vi "gm_measuringmode.vi"(9 "rt_vars in":T2, 10 "Output - Cluster gas in":T1 {"GM TS-2[°C]" format="%.2g"; "GM TS-1 [°C]" format="%.2g"; "GM DS-1 [bar]" format="%.4g"; "GM DS-2 [bar]" format="%.4g"; "GA1 h2 [%]" format="%.2g"; "GA1 co2 [%]" format="%.2g"; "GA1 ch4 [%]" format="%.2g"}, 11 "Input - Cluster gas in":T3) -> (1 "rt_vars out":T2, 2 "Output - Cluster gas out":T1 {"GM TS-2[°C]" format="%.2g"; "GM TS-1 [°C]" format="%.2g"; "GM DS-1 [bar]" format="%.4g"; "GM DS-2 [bar]" format="%.4g"; "GA1 h2 [%]" format="%.2g"; "GA1 co2 [%]" format="%.2g"; "GA1 ch4 [%]" format="%.2g"}, 3 "Input - Cluster gas out":T3)   [LabVIEW 2011]
uses:
  Input - Cluster gas.ctl
  Output - Cluster gas.ctl
panel:
  # "converted bool array!"
  # "mode :\n0: nothing\n1: quality\n2: quantity\n3: quality and quantity"
  # "converted bool array!"
  # "mode :\n0: nothing\n1: quality\n2: quantity\n3: quality and quantity"
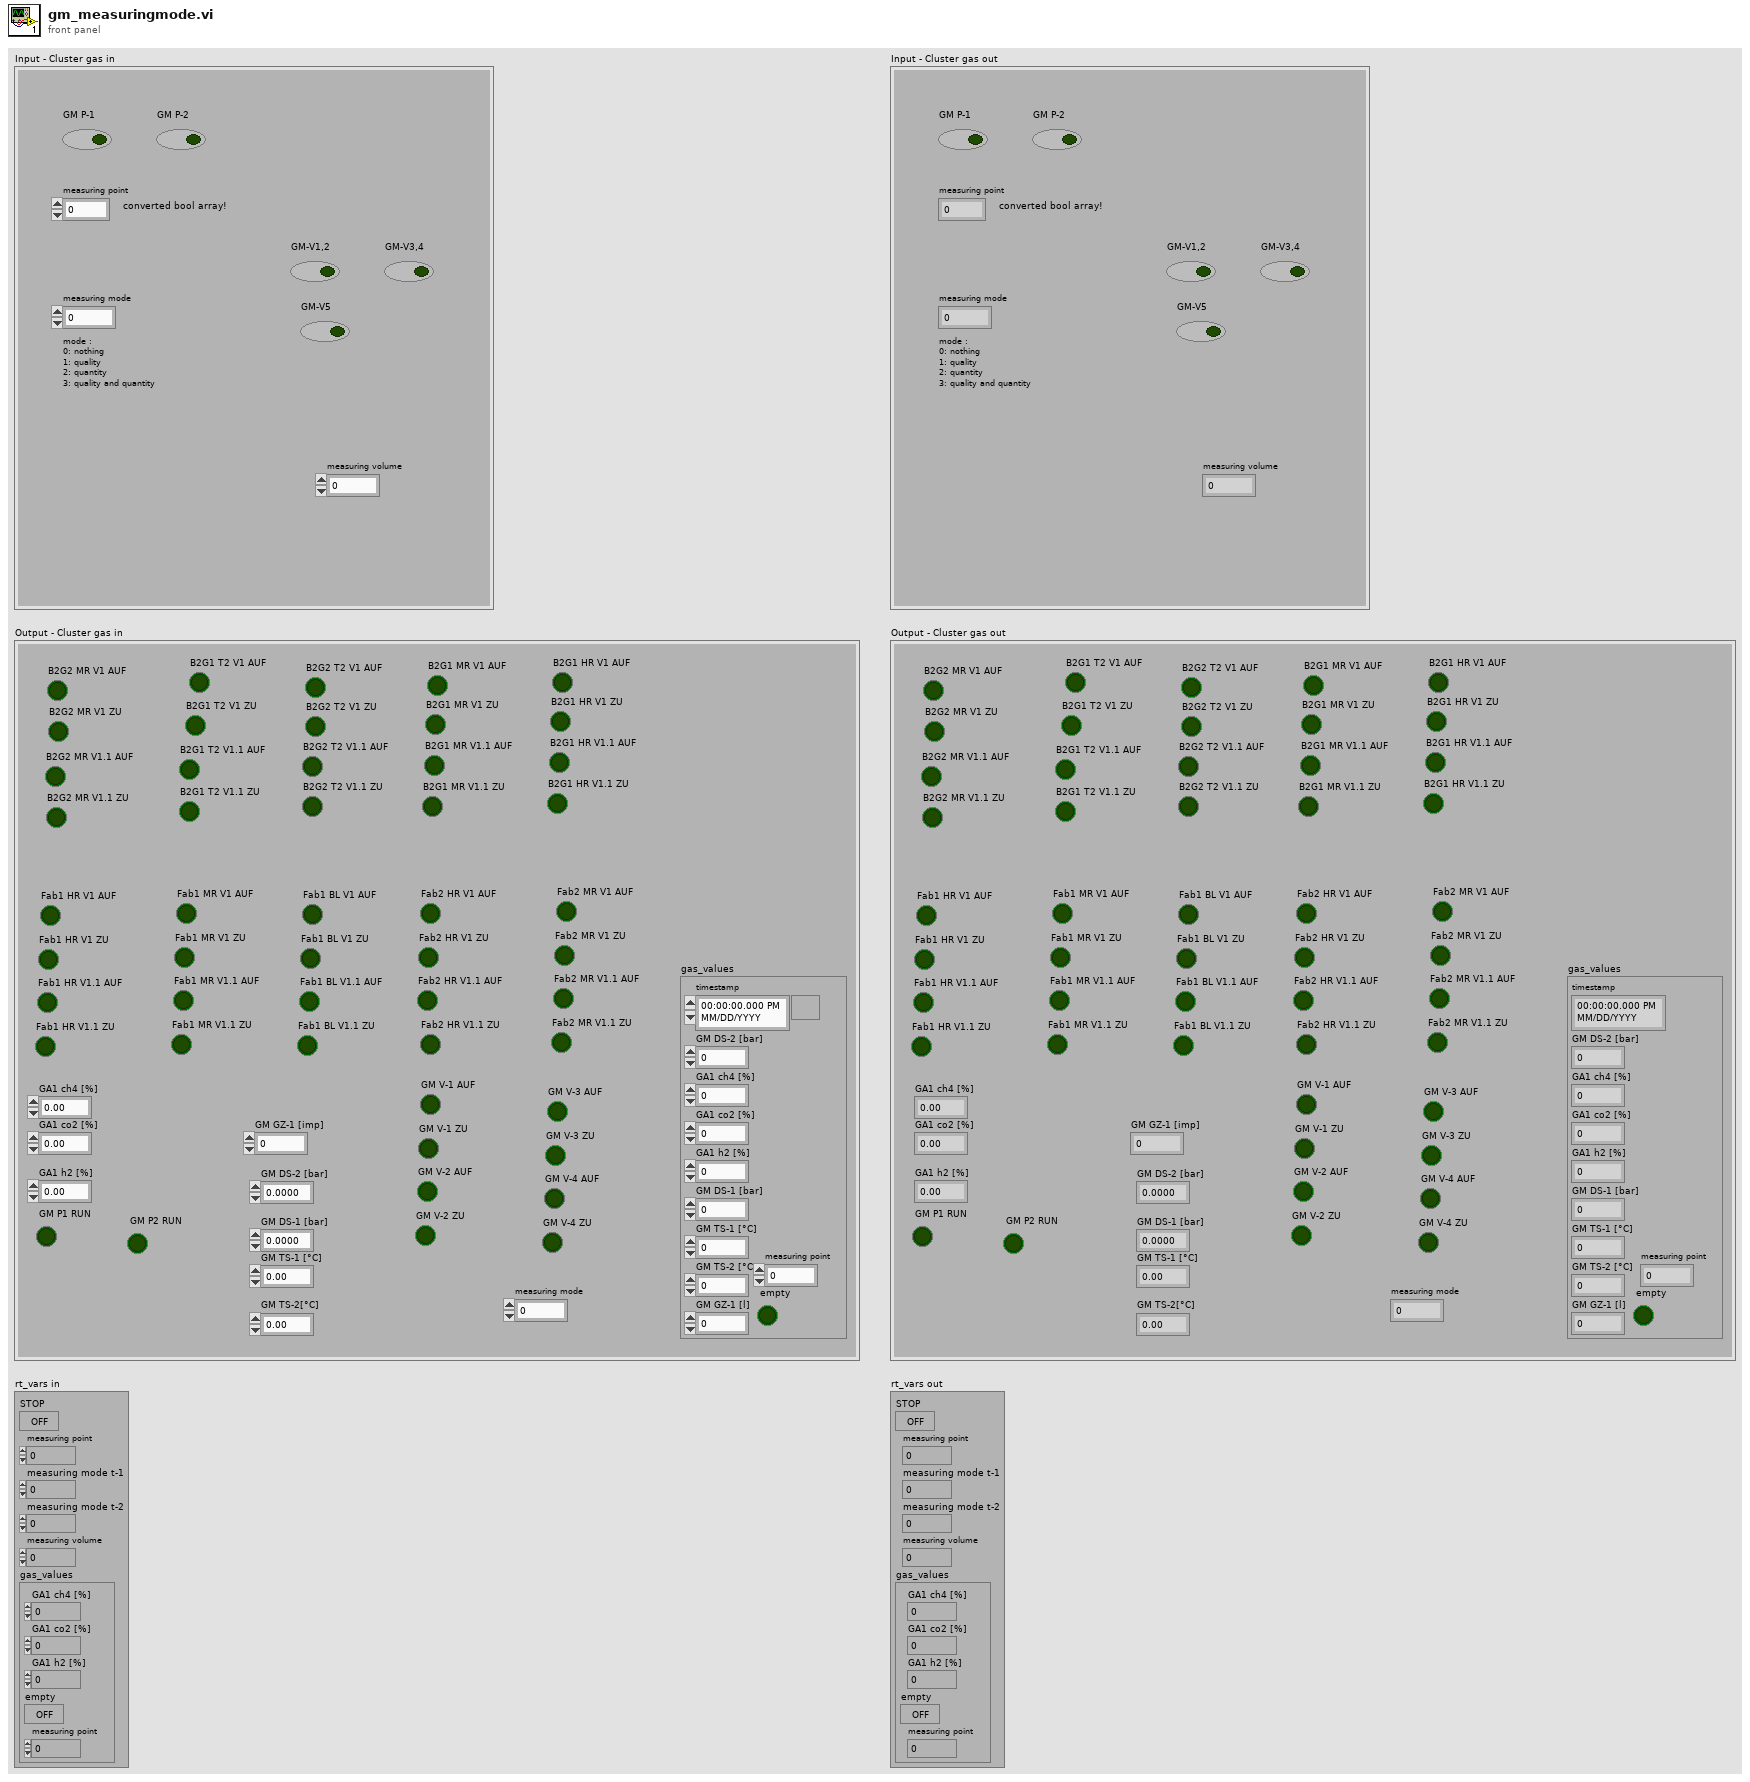
[diagram p1: front panel]
types:
  T1 = typedef "Output - Cluster gas.ctl" = cluster{"B2G2 MR V1.1 AUF":bool, "B2G2 MR V1.1 ZU":bool, "B2G2 MR V1 AUF":bool, "B2G2 MR V1 ZU":bool, "B2G1 T2 V1 AUF":bool, "B2G1 T2 V1 ZU":bool, "B2G1 T2 V1.1 AUF":bool, "B2G1 T2 V1.1 ZU":bool, "B2G2 T2 V1 AUF":bool, "B2G2 T2 V1 ZU":bool, "B2G2 T2 V1.1 ZU":bool, "B2G2 T2 V1.1 AUF":bool, "B2G1 MR V1 AUF":bool, "B2G1 MR V1 ZU":bool, "B2G1 MR V1.1 AUF":bool, "B2G1 MR V1.1 ZU":bool, "B2G1 HR V1 AUF":bool, "B2G1 HR V1 ZU":bool, "B2G1 HR V1.1 AUF":bool, "B2G1 HR V1.1 ZU":bool, "Fab1 HR V1 AUF":bool, "Fab1 HR V1 ZU":bool, "Fab1 HR V1.1 AUF":bool, "Fab1 HR V1.1 ZU":bool, "Fab1 MR V1 AUF":bool, "Fab1 MR V1 ZU":bool, "Fab1 MR V1.1 AUF":bool, "Fab1 MR V1.1 ZU":bool, "Fab1 BL V1 AUF":bool, "Fab1 BL V1 ZU":bool, "Fab1 BL V1.1 AUF":bool, "Fab1 BL V1.1 ZU":bool, "Fab2 HR V1 AUF":bool, "Fab2 HR V1 ZU":bool, "Fab2 HR V1.1 AUF":bool, "Fab2 HR V1.1 ZU":bool, "Fab2 MR V1 AUF":bool, "Fab2 MR V1 ZU":bool, "Fab2 MR V1.1 AUF":bool, "Fab2 MR V1.1 ZU":bool, "GA1 ch4 [%]":dbl, "GA1 co2 [%]":dbl, "GA1 h2 [%]":dbl, "GM P1 RUN":bool, "GM V-1 AUF":bool, "GM V-1 ZU":bool, "GM V-2 AUF":bool, "GM V-2 ZU":bool, "GM V-3 AUF":bool, "GM V-3 ZU":bool, "GM V-4 AUF":bool, "GM V-4 ZU":bool, "GM P2 RUN":bool, "GM GZ-1 [imp]":u32, "GM DS-2 [bar]":dbl, "GM DS-1 [bar]":dbl, "GM TS-1 [°C]":dbl, "GM TS-2[°C]":dbl, "gas_values":cluster{"timestamp":timestamp, "GM DS-2 [bar]":dbl, "GA1 ch4 [%]":dbl, "GA1 co2 [%]":dbl, "GA1 h2 [%]":dbl, "GM DS-1 [bar]":dbl, "GM TS-1 [°C]":dbl, "GM TS-2 [°C]":dbl, "GM GZ-1 [l]":dbl, "empty":bool, "measuring point":u8}, "measuring mode":u8}
  T2 = cluster{"STOP":bool, "measuring point":u32, "measuring mode t-1":u8, "measuring mode t-2":u8, "measuring volume":u32, "gas_values":cluster{"GA1 ch4 [%]":dbl, "GA1 co2 [%]":dbl, "GA1 h2 [%]":dbl, "empty":bool, "measuring point":u8}}
  T3 = typedef "Input - Cluster gas.ctl" = cluster{"GM P-1":bool, "GM P-2":bool, "measuring point":u32, "measuring mode":u8, "GM-V1,2":bool, "GM-V3,4":bool, "GM-V5":bool, "measuring volume":u32}
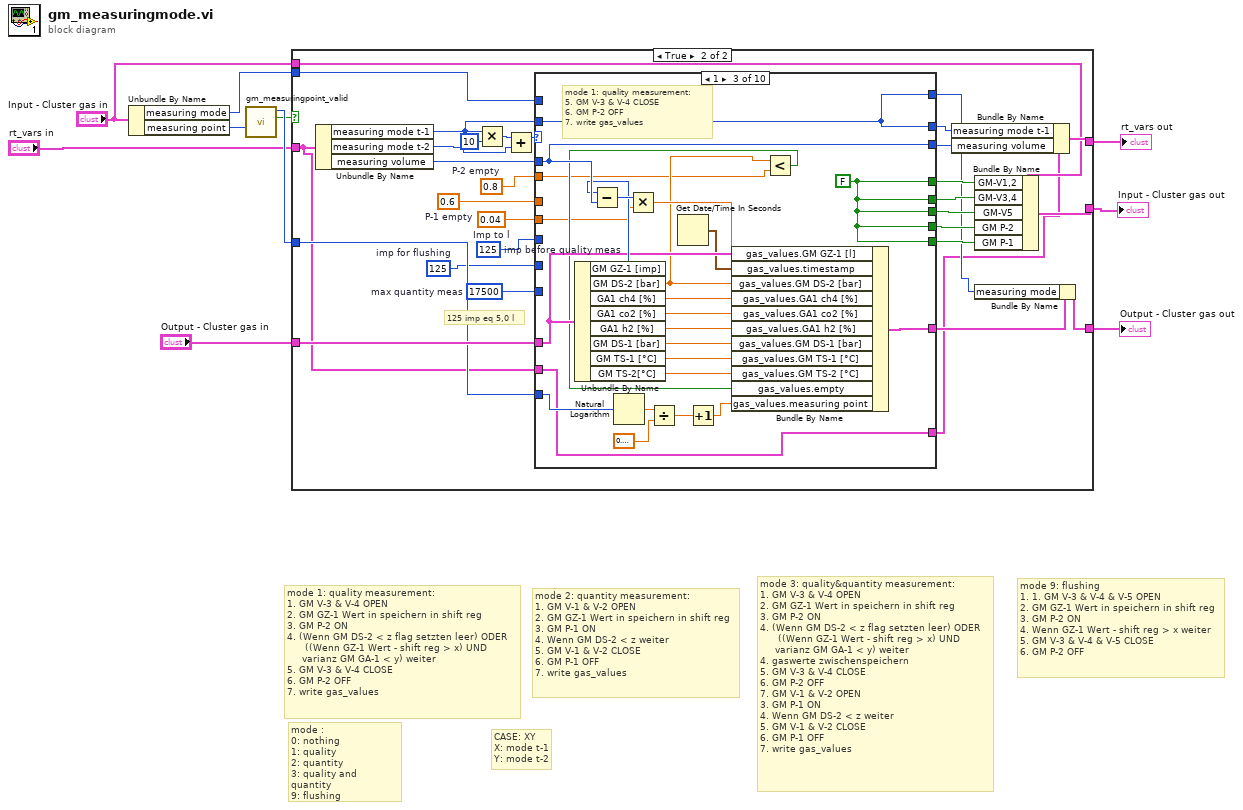
[diagram p0: block diagram]
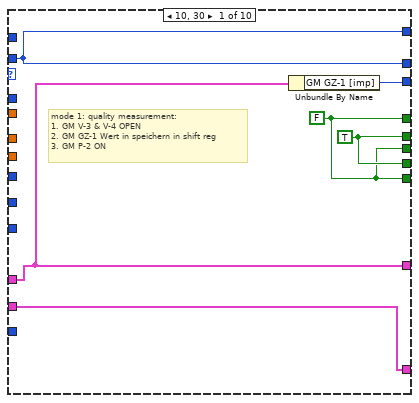
[diagram p3: hidden frame]
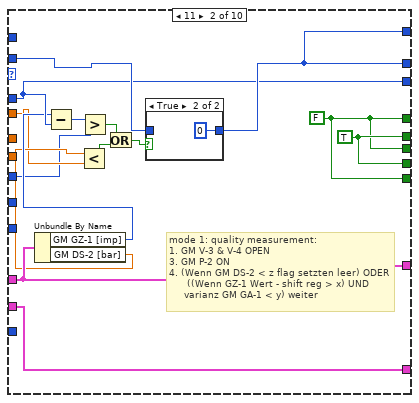
[diagram p4: hidden frame]
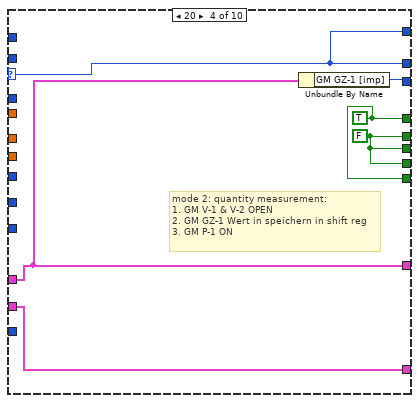
[diagram p6: hidden frame]
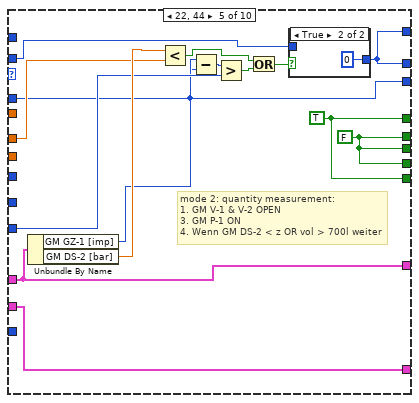
[diagram p7: hidden frame]
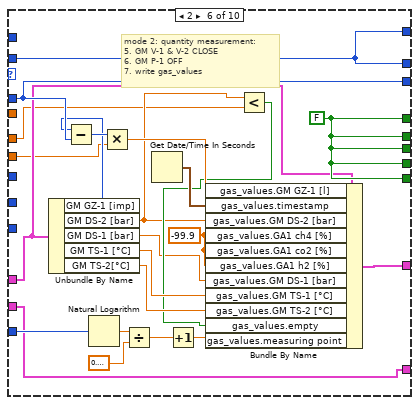
[diagram p9: hidden frame]
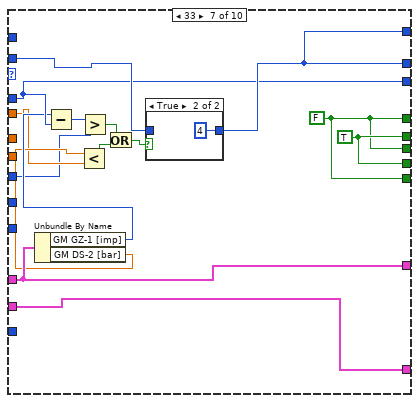
[diagram p10: hidden frame]
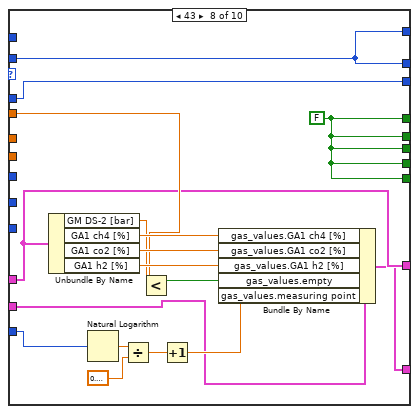
[diagram p12: hidden frame]
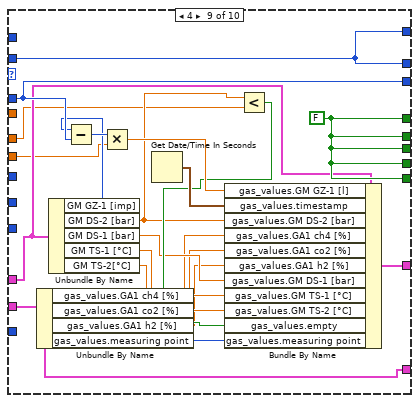
[diagram p13: hidden frame]
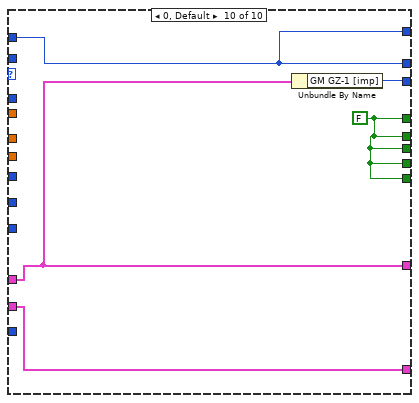
[diagram p14: hidden frame]
diagram:
  # "mode :\n0: nothing\n1: quality\n2: quantity\n3: quality and quantity\n9: flushing"
  # "mode 9: flushing\n1. 1. GM V-3 & V-4 & V-5 OPEN\n2. GM GZ-1 Wert in speichern in shift reg\n3. GM P-2 ON\n4. Wenn GZ-1 Wert - shift reg > x weiter \n5. GM V-3 & V-4 & V-5 CLOSE\n6. GM P-2 OFF"
  # "CASE: XY\nX: mode t-1\nY: mode t-2"
  # "mode 3: quality&quantity measurement:\n1. GM V-3 & V-4 OPEN\n2. GM GZ-1 Wert in speichern in shift reg\n3. GM P-2 ON\n4. (Wenn GM DS-2 < z flag setzten leer) ODER\n      ((Wenn GZ-1 Wert - shift reg > x) UND\n     varianz GM GA-1 < y) weiter\n4. gaswerte zwischenspeichern\n5. GM V-3 & V-4 CLOSE\n6. GM P-2 OFF\n7. GM V-1 & V-2 OPEN\n3. GM P-1 ON\n4. Wenn GM DS-2 < z weiter\n5. GM V-1 & V-2 CLOSE\n6. GM P-1 OFF\n7. write gas_values"
  # "mode 2: quantity measurement:\n1. GM V-1 & V-2 OPEN\n2. GM GZ-1 Wert in speichern in shift reg\n3. GM P-1 ON\n4. Wenn GM DS-2 < z weiter\n5. GM V-1 & V-2 CLOSE\n6. GM P-1 OFF\n7. write gas_values"
  # "mode 1: quality measurement:\n1. GM V-3 & V-4 OPEN\n2. GM GZ-1 Wert in speichern in shift reg\n3. GM P-2 ON\n4. (Wenn GM DS-2 < z flag setzten leer) ODER\n      ((Wenn GZ-1 Wert - shift reg > x) UND\n     varianz GM GA-1 < y) weiter\n5. GM V-3 & V-4 CLOSE\n6. GM P-2 OFF\n7. write gas_values"
  n1 = Unbundle By Name("Input - Cluster gas in") -> ("measuring mode"=w3:u8, "measuring point"=w2:u32)
  n2 = call "gm_measuringpoint_valid.vi"("measuring point in"=w2) -> ("Boolean"=w1:bool, "measuring point out"=w10:u32)  [unwired: 9 in]
  n3 = case shown="True" w1 {
    tunnel: w3 -> [_ w43]
    tunnel: "Output - Cluster gas in" -> [w13 w39]
    tunnel: [w13 w24] -> w5
    tunnel: "rt_vars in" -> [w12 w16]
    tunnel: [w12 w35] -> w7
    tunnel: "Input - Cluster gas in" -> [w11 w27]
    tunnel: [w11 w26] -> w9
    tunnel: w10 -> [_ w22]
    frame False {
    }
    frame True {
      w14 = u32 125  # imp for flushing
      w17 = u32 17500  # max quantity meas
      w18 = u32 125  # imp before quality meas
      w19 = 0.6  # P-1 empty
      w20 = 0.8  # P-2 empty
      w21 = 0.04  # Imp to l
      # "125 imp eq 5,0 l"
      n4 = Unbundle By Name(w16) -> ("measuring mode t-1"=w38:u8, "measuring mode t-2"=w37:u8, "measuring volume"=w36:u32)
      n5 = Multiply(x=w38, y=u8 10) -> (x*y=w42:u8)
      n6 = Add(x=w42, y=w37) -> (x+y=w41:u8)
      n7 = case shown="1" w41 {
        selector: w41 -> [_ _ _ w97 _ _ _ _ _ _]
        tunnel: w43 -> [_ _ _ _ _ _ _ _ _ w197]
        tunnel: [w48 w61 w90 w97 w110 w136 w149 w170 w191 w197] -> w34
        tunnel: [w44 w63 w91 w96 w112 w137 w151 w171 w192 w196] -> w32
        tunnel: [w49 w64 w91 w95 w107 w137 w152 w171 w192 w196] -> w31
        tunnel: [w44 w63 w91 w95 w107 w137 w151 w171 w192 w196] -> w30
        tunnel: [w48 w61 w90 w97 w110 w136 w149 w170 w191 w197] -> w23
        tunnel: [w46 w60 w89 w93 w100 w135 w148 w169 w190 w194] -> w33
        tunnel: [w49 w64 w91 w95 w107 w137 w152 w171 w192 w196] -> w29
        tunnel: [w44 w63 w91 w96 w112 w137 w151 w171 w192 w196] -> w28
        tunnel: w36 -> [_ w60 w89 _ w100 w135 w148 w169 w190 _]
        tunnel: w38 -> [w48 w62 w90 _ w111 w136 w150 w170 w191 _]
        tunnel: w39 -> [w47 w55 w85 w94 w109 w131 w143 w157 w186 w195]
        tunnel: [w47 w55 w86 w94 w109 w132 w143 w157 w187 w195] -> w25
        tunnel: w22 -> [_ _ w74 _ _ w120 _ w162 _ _]
        tunnel: w21 -> [_ _ w69 _ _ w116 _ _ w177 _]
        tunnel: w20 -> [_ w52 w68 _ _ _ w140 w158 _ _]
        tunnel: w19 -> [_ _ _ _ w106 w117 _ _ w178 _]
        tunnel: w18 -> [_ w51 _ _ _ _ w139 _ _ _]
        tunnel: w17 -> [_ _ _ _ w102 _ _ _ _ _]
        tunnel: w16 -> [w45 w50 w67 w92 w98 w115 w138 w156 w176 w193]
        tunnel: [w45 w50 w67 w92 w98 w115 w138 w155 w176 w193] -> w15
        tunnel: w14 -> [_ _ _ _ _ _ _ _ _ _]
        frame 10, 30 {
          w44 = FALSE ("GM-V3,4")
          w49 = TRUE ("GM-V3,4")
          # "mode 1: quality measurement:\n1. GM V-3 & V-4 OPEN\n2. GM GZ-1 Wert in speichern in shift reg\n3. GM P-2 ON"
          n8 = Unbundle By Name(w47) -> ("GM GZ-1 [imp]"=w46:u32)
        }
        frame 11 {
          w63 = FALSE ("GM-V3,4")
          w64 = TRUE ("GM-V3,4")
          # "mode 1: quality measurement:\n1. GM V-3 & V-4 OPEN\n3. GM P-2 ON\n4. (Wenn GM DS-2 < z flag setzten leer) ODER\n      ((Wenn GZ-1 Wert - shift reg > x) UND\n     varianz GM GA-1 < y) weiter"
          n9 = Unbundle By Name(w55) -> ("GM GZ-1 [imp]"=w54:u32, "GM DS-2 [bar]"=w53:dbl)
          n10 = Subtract(x=w54, y=w60) -> (x-y=w59:u32)
          n11 = Less?(x=w53, y=w52) -> (x < y?=w56:bool)
          n12 = Greater?(x=w59, y=w51) -> (0:w57:bool)
          n13 = Or(x=w57, y=w56) -> (x .or. y?=w58:bool)
          n14 = case shown="True" w58 {
            tunnel: w62 -> [w65 _]
            tunnel: [w65 u8 0 ("measuring mode t-1")] -> w61
            frame False {
            }
            frame True {
            }
          }
        }
        frame 1 {
          w91 = FALSE ("GM-V3,4")
          # "mode 1: quality measurement:\n5. GM V-3 & V-4 CLOSE\n6. GM P-2 OFF\n7. write gas_values"
          n15 = Unbundle By Name(w85) -> ("GM GZ-1 [imp]"=w87:u32, "GM DS-2 [bar]"=w71:dbl, "GA1 ch4 [%]"=w82:dbl, "GA1 co2 [%]"=w81:dbl, "GA1 h2 [%]"=w80:dbl, "GM DS-1 [bar]"=w70:dbl, "GM TS-1 [°C]"=w79:dbl, "GM TS-2[°C]"=w78:dbl)
          n16 = Subtract(x=w87, y=w89) -> (x-y=w88:u32)
          n17 = Natural Logarithm(1:w74) -> (0:w76:dbl)
          n18 = Multiply(x=w88, y=w69) -> (x*y=w83:dbl)
          n19 = Divide(x=w76, y=0.6931471805599453) -> (x/y=w73:dbl)
          n20 = Get Date/Time In Seconds ("timestamp")() -> (seconds since 1Jan1904=w84:timestamp)
          n21 = Increment(x=w73) -> (x+1=w72:dbl)
          n22 = Less?(x=w71, y=w68) -> (x < y?=w77:bool)
          n23 = Bundle By Name(cluster=w85, "gas_values.GM GZ-1 [l]"=w83, "gas_values.timestamp"=w84, "gas_values.GM DS-2 [bar]"=w71, "gas_values.GA1 ch4 [%]"=w82, "gas_values.GA1 co2 [%]"=w81, "gas_values.GA1 h2 [%]"=w80, "gas_values.GM DS-1 [bar]"=w70, "gas_values.GM TS-1 [°C]"=w79, "gas_values.GM TS-2 [°C]"=w78, "gas_values.empty"=w77, "gas_values.measuring point"=w72) -> (w86:T1)
        }
        frame 20 {
          w95 = FALSE ("GM-V3,4")
          w96 = TRUE ("GM-V3,4")
          # "mode 2: quantity measurement:\n1. GM V-1 & V-2 OPEN\n2. GM GZ-1 Wert in speichern in shift reg\n3. GM P-1 ON"
          n24 = Unbundle By Name(w94) -> ("GM GZ-1 [imp]"=w93:u32)
        }
        frame 22, 44 {
          w112 = TRUE ("GM-V3,4")
          w107 = FALSE ("GM-V3,4")
          # "mode 2: quantity measurement:\n1. GM V-1 & V-2 OPEN\n3. GM P-1 ON\n4. Wenn GM DS-2 < z OR vol > 700l weiter"
          n25 = Unbundle By Name(w109) -> ("GM GZ-1 [imp]"=w101:u32, "GM DS-2 [bar]"=w108:dbl)
          n26 = Less?(x=w108, y=w106) -> (x < y?=w105:bool)
          n27 = Subtract(x=w101, y=w100) -> (x-y=w103:u32)
          n28 = Greater?(x=w103, y=w102) -> (0:w99:bool)
          n29 = Or(x=w105, y=w99) -> (x .or. y?=w104:bool)
          n30 = case shown="True" w104 {
            tunnel: w111 -> [w113 _]
            tunnel: [w113 u8 0 ("measuring mode t-1")] -> w110
            frame False {
            }
            frame True {
            }
          }
        }
        frame 2 {
          w125 = -99.9 ("gas_values.GA1 ch4 [%]")
          w137 = FALSE ("GM-V3,4")
          # "mode 2: quantity measurement:\n5. GM V-1 & V-2 CLOSE\n6. GM P-1 OFF\n7. write gas_values"
          n31 = Unbundle By Name(w131) -> ("GM GZ-1 [imp]"=w133:u32, "GM DS-2 [bar]"=w119:dbl, "GM DS-1 [bar]"=w118:dbl, "GM TS-1 [°C]"=w128:dbl, "GM TS-2[°C]"=w127:dbl)
          n32 = Subtract(x=w133, y=w135) -> (x-y=w134:u32)
          n33 = Natural Logarithm(1:w120) -> (0:w124:dbl)
          n34 = Multiply(x=w134, y=w116) -> (x*y=w129:dbl)
          n35 = Divide(x=w124, y=0.6931471805599453) -> (x/y=w122:dbl)
          n36 = Get Date/Time In Seconds ("timestamp")() -> (seconds since 1Jan1904=w130:timestamp)
          n37 = Increment(x=w122) -> (x+1=w121:dbl)
          n38 = Less?(x=w119, y=w117) -> (x < y?=w126:bool)
          n39 = Bundle By Name(cluster=w131, "gas_values.GM GZ-1 [l]"=w129, "gas_values.timestamp"=w130, "gas_values.GM DS-2 [bar]"=w119, "gas_values.GA1 ch4 [%]"=w125, "gas_values.GA1 co2 [%]"=w125, "gas_values.GA1 h2 [%]"=w125, "gas_values.GM DS-1 [bar]"=w118, "gas_values.GM TS-1 [°C]"=w128, "gas_values.GM TS-2 [°C]"=w127, "gas_values.empty"=w126, "gas_values.measuring point"=w121) -> (w132:T1)
        }
        frame 33 {
          w151 = FALSE ("GM-V3,4")
          w152 = TRUE ("GM-V3,4")
          n40 = Unbundle By Name(w143) -> ("GM GZ-1 [imp]"=w142:u32, "GM DS-2 [bar]"=w141:dbl)
          n41 = Subtract(x=w142, y=w148) -> (x-y=w147:u32)
          n42 = Less?(x=w141, y=w140) -> (x < y?=w144:bool)
          n43 = Greater?(x=w147, y=w139) -> (0:w145:bool)
          n44 = Or(x=w145, y=w144) -> (x .or. y?=w146:bool)
          n45 = case shown="True" w146 {
            tunnel: w150 -> [w153 _]
            tunnel: [w153 u8 4 ("measuring mode t-1")] -> w149
            frame False {
            }
            frame True {
            }
          }
        }
        frame 43 {
          w171 = FALSE ("GM-V3,4")
          n46 = Unbundle By Name(w157) -> ("GM DS-2 [bar]"=w159:dbl, "GA1 ch4 [%]"=w168:dbl, "GA1 co2 [%]"=w167:dbl, "GA1 h2 [%]"=w166:dbl)
          n47 = Natural Logarithm(1:w162) -> (0:w164:dbl)
          n48 = Divide(x=w164, y=0.6931471805599453) -> (x/y=w161:dbl)
          n49 = Less?(x=w159, y=w158) -> (x < y?=w165:bool)
          n50 = Increment(x=w161) -> (x+1=w160:dbl)
          n51 = Bundle By Name(cluster=w156, "gas_values.GA1 ch4 [%]"=w168, "gas_values.GA1 co2 [%]"=w167, "gas_values.GA1 h2 [%]"=w166, "gas_values.empty"=w165, "gas_values.measuring point"=w160) -> (w155:T2)
        }
        frame 4 {
          w192 = FALSE ("GM-V3,4")
          n52 = Unbundle By Name(w176) -> ("gas_values.GA1 ch4 [%]"=w174:dbl, "gas_values.GA1 co2 [%]"=w173:dbl, "gas_values.GA1 h2 [%]"=w172:dbl, "gas_values.measuring point"=w175:u8)
          n53 = Unbundle By Name(w186) -> ("GM GZ-1 [imp]"=w188:u32, "GM DS-2 [bar]"=w180:dbl, "GM DS-1 [bar]"=w179:dbl, "GM TS-1 [°C]"=w183:dbl, "GM TS-2[°C]"=w182:dbl)
          n54 = Subtract(x=w188, y=w190) -> (x-y=w189:u32)
          n55 = Multiply(x=w189, y=w177) -> (x*y=w184:dbl)
          n56 = Get Date/Time In Seconds ("timestamp")() -> (seconds since 1Jan1904=w185:timestamp)
          n57 = Less?(x=w180, y=w178) -> (x < y?=w181:bool)
          n58 = Bundle By Name(cluster=w186, "gas_values.GM GZ-1 [l]"=w184, "gas_values.timestamp"=w185, "gas_values.GM DS-2 [bar]"=w180, "gas_values.GA1 ch4 [%]"=w174, "gas_values.GA1 co2 [%]"=w173, "gas_values.GA1 h2 [%]"=w172, "gas_values.GM DS-1 [bar]"=w179, "gas_values.GM TS-1 [°C]"=w183, "gas_values.GM TS-2 [°C]"=w182, "gas_values.empty"=w181, "gas_values.measuring point"=w175) -> (w187:T1)
        }
        frame 0, Default {
          w196 = FALSE ("GM-V3,4")
          n59 = Unbundle By Name(w195) -> ("GM GZ-1 [imp]"=w194:u32)
        }
      }
      n60 = Bundle By Name(cluster=w15, "measuring mode t-1"=w34, "measuring volume"=w33) -> (w35:T2)
      n61 = Bundle By Name(cluster=w27, "GM-V1,2"=w32, "GM-V3,4"=w31, "GM-V5"=w30, "GM P-2"=w29, "GM P-1"=w28) -> (w26:T3)
      n62 = Bundle By Name(cluster=w25, "measuring mode"=w23) -> (w24:T1)
    }
  }
  "Input - Cluster gas out" <- w9
  "rt_vars out" <- w7
  "Output - Cluster gas out" <- w5
